vi "filtruj.vi"(4 "tab. wejœciowa":dbl[](array[numeric])) -> (1 "tab. przefiltrowana":dbl[](array[numeric]))   [LabVIEW 2014]
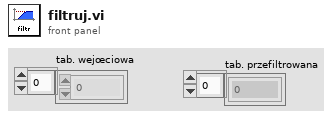
[diagram p1: front panel]
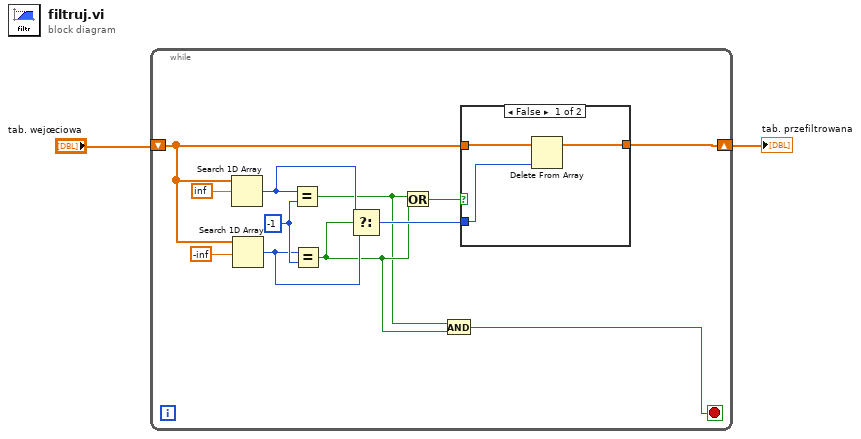
[diagram p0: block diagram]
diagram:
  n1 = while {
    shift-right: [w10] -> w1
    shift-left: "tab. wejœciowa" -> [w9]
    stop <- w3 stop-if-true
    w13 = -1 ("y")
    n2 = Search 1D Array(1D array=w9, element=inf) -> (index of element=w8:i32)  [unwired: 1 in]
    n3 = Search 1D Array(1D array=w9, element=-inf) -> (index of element=w7:i32)  [unwired: 1 in]
    n4 = Equal?(x=w8, y=w13) -> (x = y?=w4:bool)
    n5 = Equal?(x=w7, y=w13) -> (x = y?=w5:bool)
    n6 = Select(t=w8, s=w5, f=w7) -> (s? t:f=w6:i32)
    n7 = Or(x=w4, y=w5) -> (x .or. y?=w11:bool)
    n8 = And(x=w4, y=w5) -> (x .and. y?=w3:bool)
    n9 = case shown="False" w11 {
      tunnel: [w16 w18] -> w10
      tunnel: w9 -> [w17 w18]
      tunnel: w6 -> [w15 _]
      frame False {
        n10 = Delete From Array(array=w17, index=w15) -> (array with subset deleted=w16:dbl[])  [unwired: 1 in, 1 out]
      }
      frame True {
      }
    }
  }
  "tab. przefiltrowana" <- w1
